vi "SetAxisPos.vi"(1 "Position":sgl format="%.2f", 2 "Axis":i32) -> (0 "error out":errorcluster)   [LabVIEW 2009]
panel:
  in  "VI Refnum":refnum<vi>
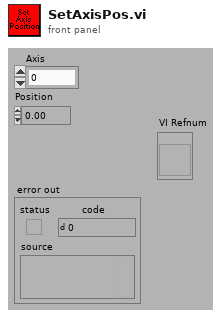
[diagram p1: front panel]
types:
  T1 = enum16{"Get Type", "Set Type", "GetStageInit", "GetWriteStageSetting", "GetInitializeStageOutput", "GetSetAxisPosition", "GetSetPos"}
  T2 = typedef "StageType.ctt" = enum16{"PI analogue", "PI 712 TCP/IP", "Märzhäuser", "PI analogue step", "PI 712 USB"}
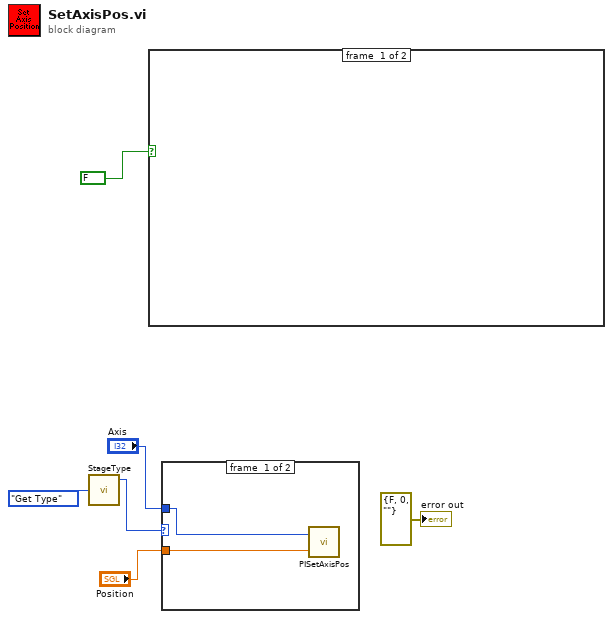
[diagram p0: block diagram]
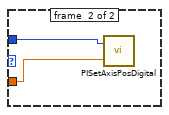
[diagram p2: hidden frame]
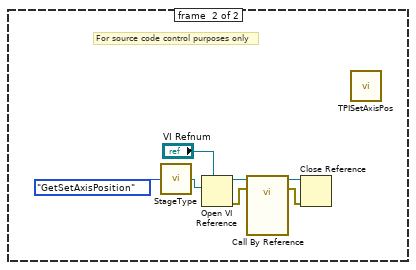
[diagram p3: hidden frame]
diagram:
  n1 = call "StageType.vi"("Function"=T1."Get Type") -> ("Stage Type (output)"=w3:T2)  [unwired: 2 in, 2 out]
  n2 = case shown="True" FALSE ("Case Constant\n(See Context Help)") {
    frame #0 {
    }
    frame #1 {
      # "For source code control purposes only"
      n3 = call "StageType.vi"("Function"=T1."GetSetAxisPosition") -> ("VI Path"=w8:path)  [unwired: 2 in, 2 out]
      n4 = Open VI Reference(type specifier VI Refnum (for type only)="VI Refnum", vi path=w8) -> (vi reference=w9:refnum<vi>, error out=w10:errorcluster)  [unwired: 4 in]
      n5 = call-by-ref "?"(reference=w9, error in=w10) -> (reference out=w11:refnum<vi>, error out=w12:errorcluster)  [unwired: 2 in]
      n6 = Close Reference(reference=w11, error in (no error)=w12) -> ()  [unwired: 1 out]
      n7 = call "TPISetAxisPos.vi"() -> ()  [unwired: 2 in]
    }
  }
  n8 = case shown="\"PI 712 TCP/IP\", \"PI 712 USB\"" w3 {
    tunnel: "Position" -> [w15 w16]
    tunnel: "Axis" -> [w14 w17]
    frame #0 {
      n9 = call "PISetAxisPos.vi"("Position"=w15, "Axis"=w14) -> ()
    }
    frame #1 {
      n10 = call "PISetAxisPosDigital.vi"("Position"=w16, "Axis"=w17) -> ()
    }
  }
  "error out" <- errorcluster {"status"=FALSE, "code"=0, "source"=""} ("error out")
